vi "USB Device Filter.vi"(9 "Device Name":string[](array[string])=["", "", "", "", "\n"], 10 "Num Dev":u32, 11 "Device Address":refnum<visa-resource-name>[](array[refnum])) -> (1 "Device Name 2":string[](array[string])=["", "", "", "", "\n"], 2 "Num Dev 2":u32, 3 "Device Address 2":refnum<visa-resource-name>[](array[refnum]))   [LabVIEW 2020]
panel:
  in  "VISA resource name out":refnum<visa-resource-name>
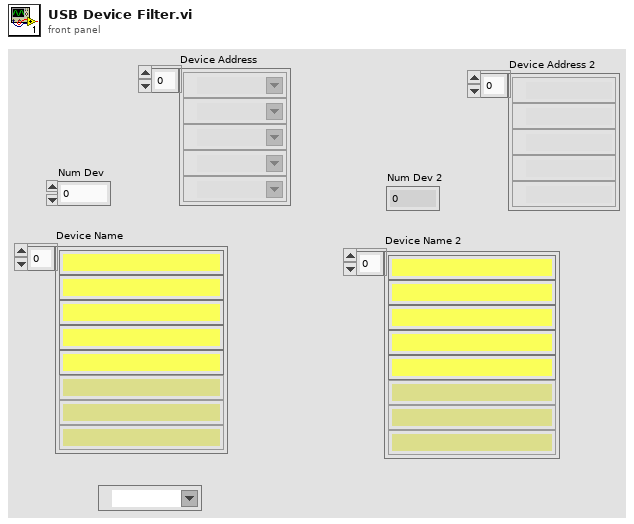
[diagram p1: front panel]
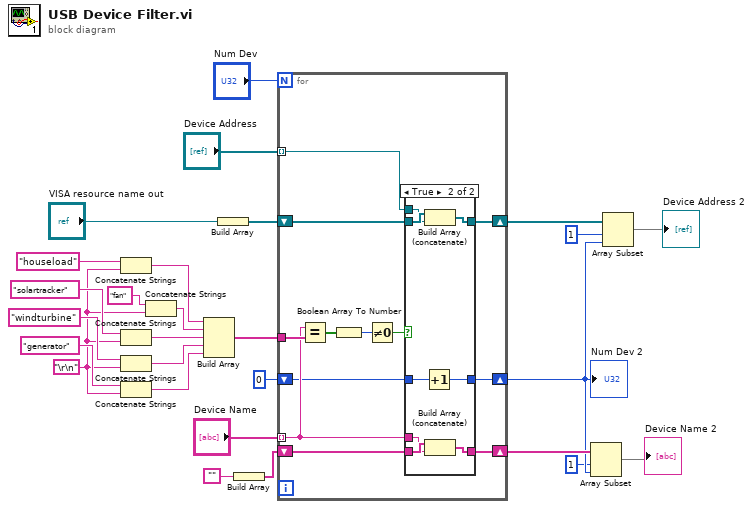
[diagram p0: block diagram]
diagram:
  w12 = "\r\n"
  n1 = Concatenate Strings("houseload", w12) -> (w21:string)
  n2 = Concatenate Strings("solartracker", w12) -> (w17:string)
  n3 = Concatenate Strings("windturbine", w12) -> (w15:string)
  n4 = Concatenate Strings("generator", w12) -> (w13:string)
  n5 = Concatenate Strings("fan", w12) -> (w19:string)
  n6 = Build Array(w21, w19, w17, w15, w13) -> (w25:string[])
  n7 = Build Array("VISA resource name out") -> (w8:refnum<visa-resource-name>[])
  n8 = Build Array("") -> (w10:string[])
  n9 = for {
    N: "Num Dev" -> [_]
    tunnel: "Device Address" -> [w32] mode=indexing
    tunnel: "Device Name" -> [w36] mode=indexing
    tunnel: w25 -> [w39]
    shift-right: [w33] -> w4
    shift-left: w10 -> [w34]
    shift-right: [w30] -> w7
    shift-left: w8 -> [w31]
    shift-right: [w28] -> w3
    shift-left: 0 -> [w29]
    n10 = Equal?(x=w36, y=w39) -> (x = y?=w38:bool[])
    n11 = Boolean Array To Number(Boolean array=w38) -> (number=w37:u32)
    n12 = Not Equal To 0?(x=w37) -> (x != 0?=w35:bool)
    n13 = case shown="True" w35 {
      tunnel: w36 -> [_ w43]
      tunnel: w34 -> [w42 w44]
      tunnel: [w42 w50] -> w33
      tunnel: w32 -> [_ w45]
      tunnel: [w41 w49] -> w30
      tunnel: w31 -> [w41 w46]
      tunnel: w29 -> [w40 w48]
      tunnel: [w40 w47] -> w28
      frame False {
      }
      frame True {
        n14 = Increment(x=w48) -> (x+1=w47:i32)
        n15 = Build Array (concatenate)(w46, w45) -> (w49:refnum<visa-resource-name>[])
        n16 = Build Array (concatenate)(w44, w43) -> (w50:string[])
      }
    }
  }
  "Num Dev 2" <- w3
  n17 = Array Subset(array=w4, index=1, length=w3) -> (→"Device Name 2":string[])
  n18 = Array Subset(array=w7, index=1, length=w3) -> (→"Device Address 2":refnum<visa-resource-name>[])
